vi "Benchmark SV Send  LV2012 - NI Verified - 2.vi"() -> ()   [LabVIEW 2015]
uses:
  <vilib>/Platform/TimedLoop/XDataNode/timing_clust.ctl
  <vilib>/Platform/TimedLoop/XDataNode/nitl_modes.ctl
  <vilib>/Platform/TimedLoop/XDataNode/wakeup.ctl
  <vilib>/platform/TimedLoop/XDataNode/XDataNode.xnode
  <vilib>/Platform/TimedLoop/XDataNode/XDNodeRunTimeDep.lvlib
panel:
  in  "Period":i64
  out "MirrorCoverMotor 2":T1
  out "appended array":dbl[](array[numeric])
  in  "Status":string[](array[string])=["Close", "Close", "Close", "Close", "Close", "Close", "Close", "Close"]
  in  "Brake Voltage FB":bool[](array[boolean])=[FALSE, FALSE, FALSE, FALSE, FALSE, TRUE, TRUE, TRUE]
  in  "Motor Voltage FB":bool[](array[boolean])=[FALSE, FALSE, FALSE, FALSE, FALSE, FALSE, FALSE, TRUE]
  in  "Brake":bool[](array[boolean])=[FALSE, FALSE, FALSE, FALSE, FALSE, FALSE, FALSE, TRUE]
  in  "Direction":bool[](array[boolean])=[FALSE, FALSE, FALSE, FALSE, FALSE, FALSE, FALSE, TRUE]
  in  "Enable":bool[](array[boolean])=[FALSE, FALSE, FALSE, FALSE, FALSE, FALSE, FALSE, TRUE]
  in  "Reset":bool
  out "Tries":u32
  out "Average Delay (ms)":dbl
  out "Delay (ms)":u32
  in  "stop":bool
  # "Overview:  Coding that exemplifies how to benchmark the communication of Shared Variables.\nRequirements: LabVIEW 2012 or compatible\nInstructions:\n1.  Run the \"Benchmark SV Receive LV2012 - NI Verified.vi\"\n2. Run this VI\n3. Watch the amount of time it takes to communicate\n4. Stop both VIs"
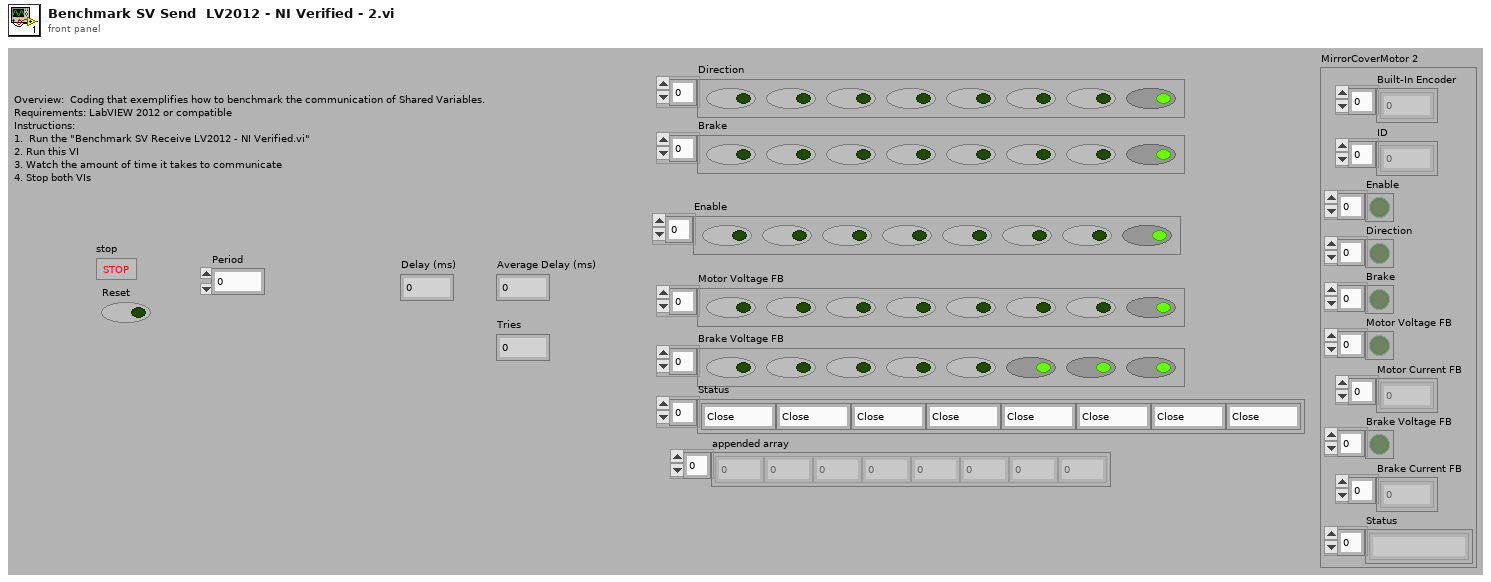
[diagram p1: front panel]
types:
  T1 = cluster{"Built-In Encoder":i32[], "ID":i16[], "Enable":bool[], "Direction":bool[], "Brake":bool[], "Motor Voltage FB":bool[], "Motor Current FB":i32[], "Brake Voltage FB":bool[], "Brake Current FB":i32[], "Status":string[]}
  T2 = typedef "XDNodeRunTimeDep.lvlib/timing_clust.ctl" = cluster{"Expected End [f-1]":u64, "Actual End [f-1]":u64, "Finished Late? [f-1]":bool, "Expected End [i-1]":u64, "Actual End [i-1]":u64, "Finished Late? [i-1]":bool, "Expected Start [i]":u64, "Actual Start [i]":u64, "Expected Start [f]":u64, "Actual Start [f]":u64, "Source Name":string, "Structure Name":string, "Period":i64, "Deadline":i64, "Offset":i64, "Start":i64, "Priority":i32, "Timeout":i32, "Mode":T3, "Wakeup Reason":T4, "Error":errorcluster, "Source Type":string, "Secondary Source Type":string, "Global End Time":u64, "Global Start Time":u64, "Frame Duration":u64, "Iteration Duration":u64, "Assigned CPU":i32, "I/O Scan Engine Mode":u32}
  T3 = typedef "XDNodeRunTimeDep.lvlib/nitl_modes.ctl" = enum32{"No Change", "Process missed periods, maintain original phase", "Discard missed periods, maintain original phase", "Process missed periods, ignore original phase", "Discard missed periods, ignore original phase"}
  T4 = typedef "XDNodeRunTimeDep.lvlib/wakeup.ctl" = enum32{"Normal", "Aborted", "Asynchronous wakeup", "Timing source error", "Timed loop error", "Timeout"}
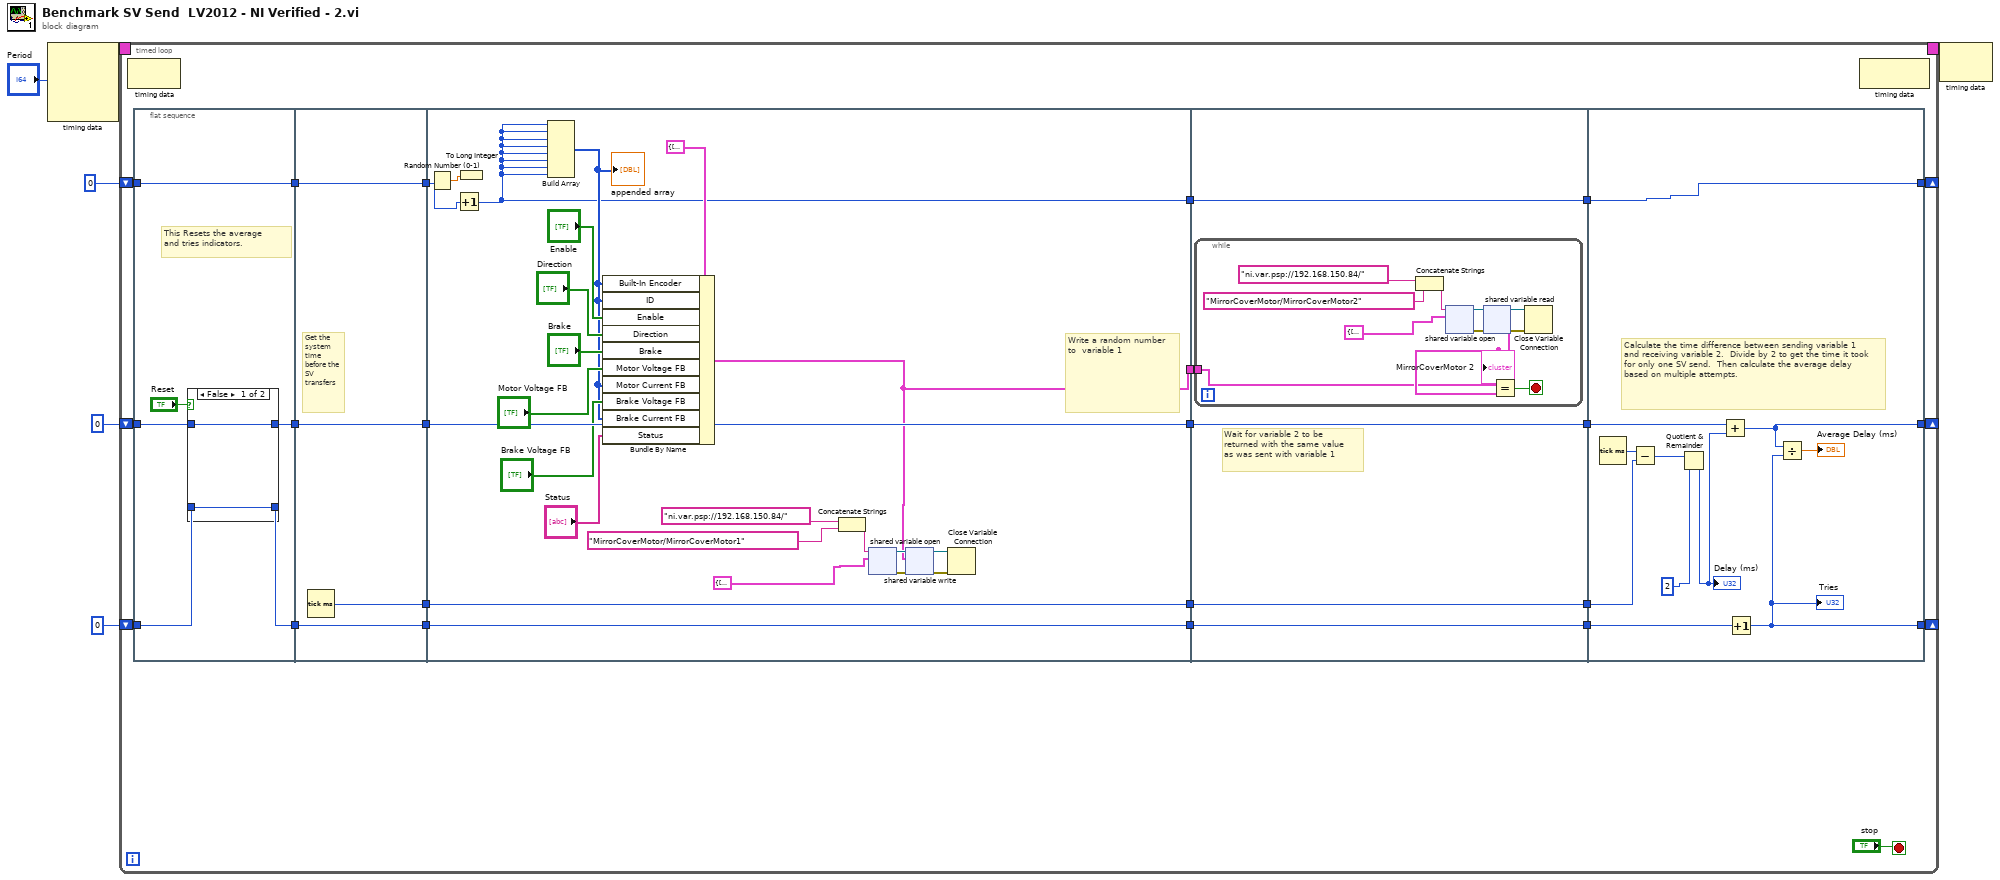
[diagram p0: block diagram]
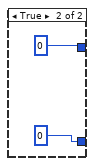
[diagram p2: hidden frame]
diagram:
  n1 = node-c288("Period") -> (w3:T2)  [unwired: 3 in]
  n2 = timed-loop {
    shift-right: [w25] -> _
    shift-left: u32 0 -> [w13]
    shift-right: [w22] -> _
    shift-left: u32 0 -> [w14]
    shift-right: [w7] -> _
    shift-left: u32 0 -> [w10]
    timing: w3 -> [_]
    timing-out: [_] -> w2
    stop <- "stop" stop-if-true
    n3 = node-c288() -> ()  [unwired: 1 in, 1 out]
    n4 = flat-sequence {
      tunnel: w13 -> [w37]
      tunnel: [w36] -> w18
      tunnel: [w34] -> w16
      tunnel: w14 -> [w33]
      tunnel: [w32] -> w11
      tunnel: w10 -> [w32]
      tunnel: [w43] -> w19
      tunnel: w18 -> [w45]
      tunnel: [w45] -> w17
      tunnel: w16 -> [w44]
      tunnel: [w44] -> w15
      tunnel: [w42] -> w12
      tunnel: w11 -> [w42]
      tunnel: [w49] -> w28
      tunnel: [w68] -> w27
      tunnel: [w67] -> w23
      tunnel: [w66] -> w20
      tunnel: w19 -> [w68]
      tunnel: w17 -> [w67]
      tunnel: w15 -> [w66]
      tunnel: w12 -> [w47]
      tunnel: [w46] -> w8
      tunnel: w28 -> [w73]
      tunnel: [w72] -> w26
      tunnel: w27 -> [w72]
      tunnel: [w71] -> w24
      tunnel: w23 -> [w71]
      tunnel: [w70] -> w21
      tunnel: w20 -> [w70]
      tunnel: [w69] -> w9
      tunnel: w8 -> [w69]
      tunnel: w26 -> [w94]
      tunnel: [w87] -> w25
      tunnel: w24 -> [w89]
      tunnel: [w86] -> w22
      tunnel: w21 -> [w93]
      tunnel: w9 -> [w85]
      tunnel: [w85] -> w7
      frame #0 {
        # "This Resets the average \nand tries indicators."
        n5 = case shown="False" "Reset" {
          tunnel: [w39 u32 0] -> w36
          tunnel: w37 -> [w39 _]
          tunnel: [w38 u32 0] -> w34
          tunnel: w33 -> [w38 _]
          frame False {
          }
          frame True {
          }
        }
      }
      frame #1 {
        # "Get the system time before the SV transfers"
        n6 = Tick Count (ms)() -> (millisecond timer value=w43:u32)
      }
      frame #2 {
        # "Write a random number to  variable 1"
        n7 = Random Number (0-1)() -> (number: 0 to 1=w48:dbl)
        n8 = Increment(x=w47) -> (x+1=w46:u32)
        n9 = To Long Integer(number=w48) -> ()  [unwired: 1 out]
        n10 = Build Array(w46, w46, w46, w46, w46, w46, w46, w46) -> (w53:u32[])
        "appended array" <- w53
        n11 = Bundle By Name(cluster=T1 {"Built-In Encoder"=[], "ID"=[], "Enable"=[], "Direction"=[], "Brake"=[], "Motor Voltage FB"=[], "Motor Current FB"=[], "Brake Voltage FB"=[], "Brake Current FB"=[], "Status"=[]} ("input cluster"), "Built-In Encoder"=w53, "ID"=w53, "Enable"="Enable", "Direction"="Direction", "Brake"="Brake", "Motor Voltage FB"="Motor Voltage FB", "Motor Current FB"=w53, "Brake Voltage FB"="Brake Voltage FB", "Brake Current FB"=w53, "Status"="Status") -> (w49:T1)
        n12 = Concatenate Strings("ni.var.psp://192.168.150.84/" ("string"), "MirrorCoverMotor/MirrorCoverMotor1") -> (w61:string)
        n13 = shared-variable-open(w61, T1 {"Built-In Encoder"=[], "ID"=[], "Enable"=[], "Direction"=[], "Brake"=[], "Motor Voltage FB"=[], "Motor Current FB"=[], "Brake Voltage FB"=[], "Brake Current FB"=[], "Status"=[]} ("MirrorCoverMotor")) -> (w65:refnum<k21>, w62:errorcluster)  [unwired: 2 in]
        n14 = shared-variable-write(w65, w62, w49) -> (w63:refnum<k21>, w64:errorcluster)
        n15 = Close Variable Connection(8:w64, 11:w63) -> ()  [unwired: 1 out]
      }
      frame #3 {
        # "Wait for variable 2 to be returned with the same value as was sent with variable 1"
        n16 = while {
          tunnel: w73 -> [w74]
          stop <- w84 stop-if-true
          n17 = Concatenate Strings("ni.var.psp://192.168.150.84/" ("string"), "MirrorCoverMotor/MirrorCoverMotor2") -> (w82:string)
          n18 = shared-variable-open(w82, T1 {"Built-In Encoder"=[], "ID"=[], "Enable"=[], "Direction"=[], "Brake"=[], "Motor Voltage FB"=[], "Motor Current FB"=[], "Brake Voltage FB"=[], "Brake Current FB"=[], "Status"=[]} ("MirrorCoverMotor")) -> (w78:refnum<k21>, w81:errorcluster)  [unwired: 2 in]
          n19 = shared-variable-read(w78, w81) -> (w80:refnum<k21>, w79:errorcluster, w77:T1)  [unwired: 1 out]
          "MirrorCoverMotor 2" <- w77
          n20 = Equal?(x=w74, y=w77) -> (x = y?=w84:bool)
          n21 = Close Variable Connection(8:w79, 11:w80) -> ()  [unwired: 1 out]
        }
      }
      frame #4 {
        # "Calculate the time difference between sending variable 1 and receiving variable 2.  Divide by 2 to get the time it took for only one SV send.  Then calculate the average delay based on multiple attempts."
        n22 = Tick Count (ms)() -> (millisecond timer value=w95:u32)
        n23 = Subtract(x=w95, y=w94) -> (x-y=w92:u32)
        n24 = Quotient & Remainder(x=w92, y=u32 2) -> (floor(x/y)=w90:u32)  [unwired: 1 out]
        "Delay (ms)" <- w90
        n25 = Add(x=w89, y=w90) -> (x+y=w87:u32)
        n26 = Increment(x=w93) -> (x+1=w86:u32)
        "Tries" <- w86
        n27 = Divide(x=w87, y=w86) -> (x/y=→"Average Delay (ms)":dbl)
      }
    }
    n28 = node-c288() -> ()  [unwired: 1 in, 1 out]
  }
  n29 = node-c288(w2) -> ()  [unwired: 1 out]
